vi "FT_Set_Flow_Control.vi"(7 "XOff":u8 format="%x", 8 "error in":errorcluster, 9 "XOn":u8 format="%x", 10 "Flow Control":u16(ring) items=["None"=0, "RTS-CTS"=256, "DTR-DSR"=512, "XOn-XOff"=1024], 11 "Handle":u32) -> (0 "error out":errorcluster, 3 "Handle out":u32)   [LabVIEW 2016]
uses:
  FTD2XX.dll
panel:
  # "Set flow control\n\nFlow control = 0x0000, 0x0100, 0x0200 or 0x0400"
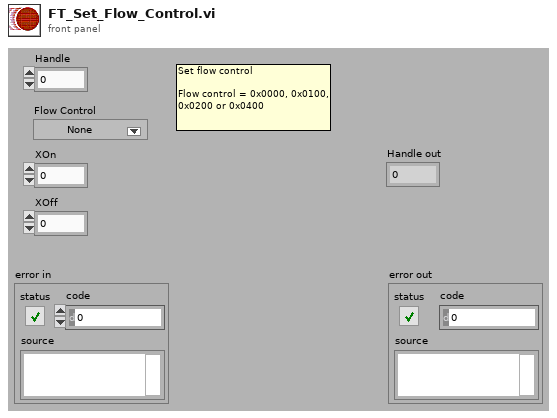
[diagram p1: front panel]
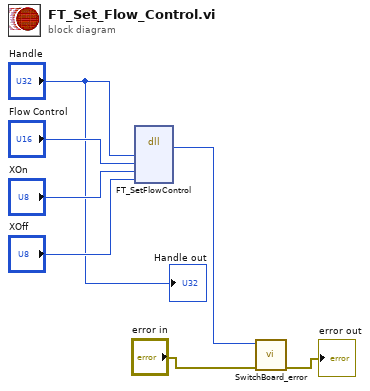
[diagram p0: block diagram]
diagram:
  n1 = dll-call lib="FTD2XX.dll" fn="FT_SetFlowControl"("Handle"="Handle", "FlowControl"="Flow Control", "XOn"="XOn", "XOff"="XOff") -> ("FT_Status"=w1:u32)  [unwired: 7 in, 2 out]
  n2 = call "SwitchBoard_error.vi"("error constant"="error in", "Code"=w1) -> ("error IO"=→"error out":errorcluster)  [unwired: 9 in]
  "Handle out" <- "Handle"
